vi "json Query - string path.vi"(8 "error in (no error)":errorcluster, 10 "path":string, 11 "JSON Document in":refnum<class "JSON Document.lvclass">) -> (0 "error out":errorcluster, 1 "type":T1, 2 "found?":bool, 3 "JSON Document out":refnum<class "JSON Document.lvclass">)   [LabVIEW 2015, in "JSON Document.lvclass"]
uses:
  JSON Document.lvclass
  rapidjson wrapper/jsonType.ctl
  JSON Document.lvclass/JSON Document.ctl
  rapidjson wrapper/rapidjson wrapper.lvlib
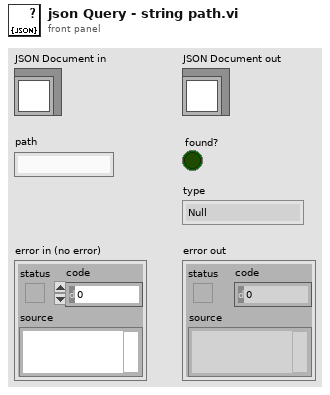
[diagram p1: front panel]
types:
  T1 = typedef "rapidjson wrapper.lvlib/jsonType.ctl" = enum16{"Null", "False", "True", "Object", "Array", "String", "Number"}
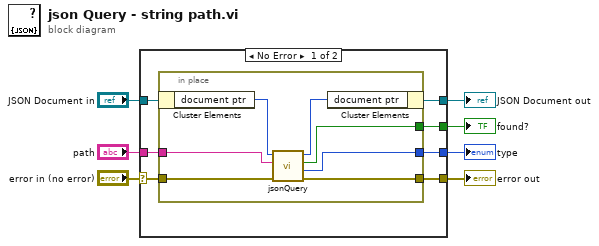
[diagram p0: block diagram]
diagram:
  n1 = case shown="No Error" "error in (no error)" {
    selector: "error in (no error)" -> [w12 w23]
    tunnel: [w11 w23] -> w6
    tunnel: [w10 w22] -> w4
    tunnel: "JSON Document in" -> [w14 w22]
    tunnel: "path" -> [w13 _]
    tunnel: [w9 _] -> w2
    tunnel: [w8 _] -> w1
    frame No Error {
      n2 = in-place {
        in-place-border: w13 -> [w19]
        in-place-border: w12 -> [w18]
        in-place-border: [w17] -> w11
        in-place-border: [w16] -> w9
        in-place-border: [w15] -> w8
        n3 = in-place-cluster #1(w14) -> ("document ptr"=w21:i64)
        n4 = call "jsonQuery.vi"("error in (no error)"=w18, "path"=w19, "d in"=w21) -> ("error out"=w17:errorcluster, "json type"=w15:T1, "found?"=w16:bool, "d out"=w20:i64)  [unwired: 5 in]
        n5 = in-place-cluster #1("document ptr"=w20) -> (w10:refnum<class "JSON Document.lvclass">)
      }
    }
    frame Error {
    }
  }
  "error out" <- w6
  "JSON Document out" <- w4
  "type" <- w1
  "found?" <- w2
